vi "Write Max RPM.vi"(8 "error in (no error)":errorcluster, 10 "Max RPM":dbl, 11 "Thruster in":refnum<class "Thruster.lvclass">) -> (0 "error out":errorcluster, 3 "Thruster out":refnum<class "Thruster.lvclass">)   [LabVIEW 2014, in "Thruster.lvclass"]
uses:
  Thruster.lvclass
  Thruster.lvclass/Thruster.ctl
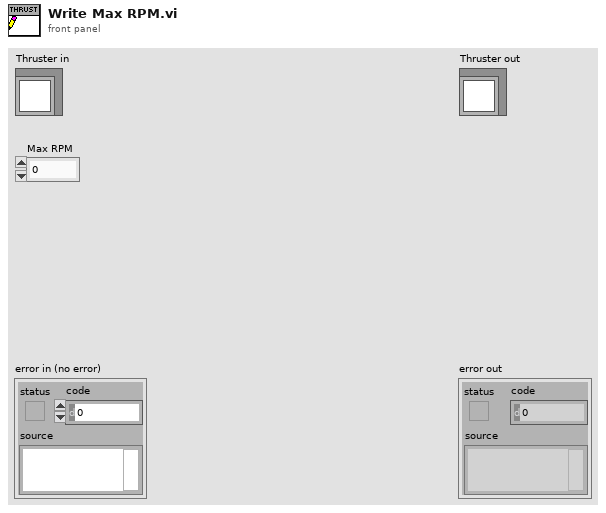
[diagram p1: front panel]
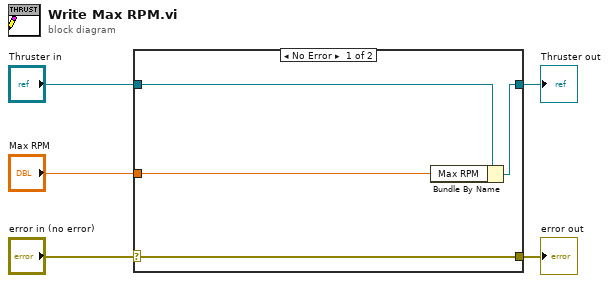
[diagram p0: block diagram]
diagram:
  n1 = case shown="No Error" "error in (no error)" {
    selector: "error in (no error)" -> [w9 w10]
    tunnel: [w9 w10] -> w4
    tunnel: [w7 w11] -> w2
    tunnel: "Thruster in" -> [w8 w11]
    tunnel: "Max RPM" -> [w6 _]
    frame No Error {
      n2 = Bundle By Name(cluster=w8, "Max RPM"=w6) -> (w7:refnum<class "Thruster.lvclass">)
    }
    frame Error {
    }
  }
  "error out" <- w4
  "Thruster out" <- w2
